vi "Send Message.vi"(0 "message queue in":T3, 1 "receiver port (0)":u16, 5 "message":T1, 9 "timeout (-1 ms)":i32=-1, 11 "error in":errorcluster) -> (4 "message queue out":T3, 10 "timed out?":bool, 15 "error out":errorcluster)   [LabVIEW 2015, in "Car Wash.lvlib" / "AMC.lvlib"]
doc: "Adds a message to:\n- the local queue passed in by reference if \"receiver host\" and \"receiver process\" are left undefined\n- another message queue on the local target if \"receiver host\" is undefined, but \"receiver process\" is specified\n- the message dispatch queue in another application instance if the receiver host and process are specified.\n\nIf \"receiver port\" is undefined, this VI will attempt to use the default UDP port.\n\nIf \"priority message\" is True, the message will be added to the front of the message queue.\n\nIf \"acknowledge message\" is True and the message is sent to another application instance, the receiver will send a reply message with the name format of \"AMC_Ack\" and a value of <name>. If \"message queue in\" is undefined, no acknowledge message will be sent."
uses:
  AMC.lvlib
  Message Queue.ctl
  Message.ctl
  Tools/Keyed Array/KeyedArray.ctl
  Send Message to Local Process.vi
  Send Message to Current Process.vi
  Read Local Dispatcher Port.vi
  FG Dispatcher Status.vi
  Get Local Name and IP.vi
  Globals.vi
  Tools/Keyed Array/Tools_KeyedArray.lvlib
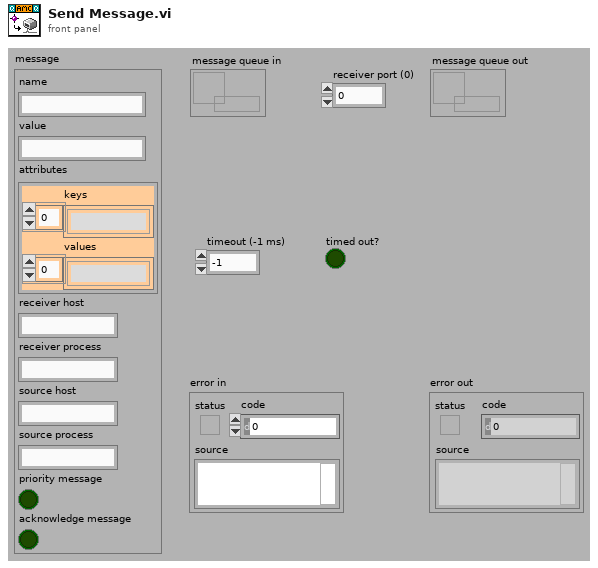
[diagram p1: front panel]
types:
  T1 = typedef "Car Wash.lvlib/AMC.lvlib/Message.ctl" = cluster{"name":string, "value":string, "attributes":T2, "receiver host":string, "receiver process":string, "source host":string, "source process":string, "priority message":bool, "acknowledge message":bool}
  T2 = typedef "Car Wash.lvlib/Tools_KeyedArray.lvlib/KeyedArray.ctl" = cluster{"keys":string[], "values":string[]}
  T3 = typedef "Car Wash.lvlib/AMC.lvlib/Message Queue.ctl" = refnum<queue>
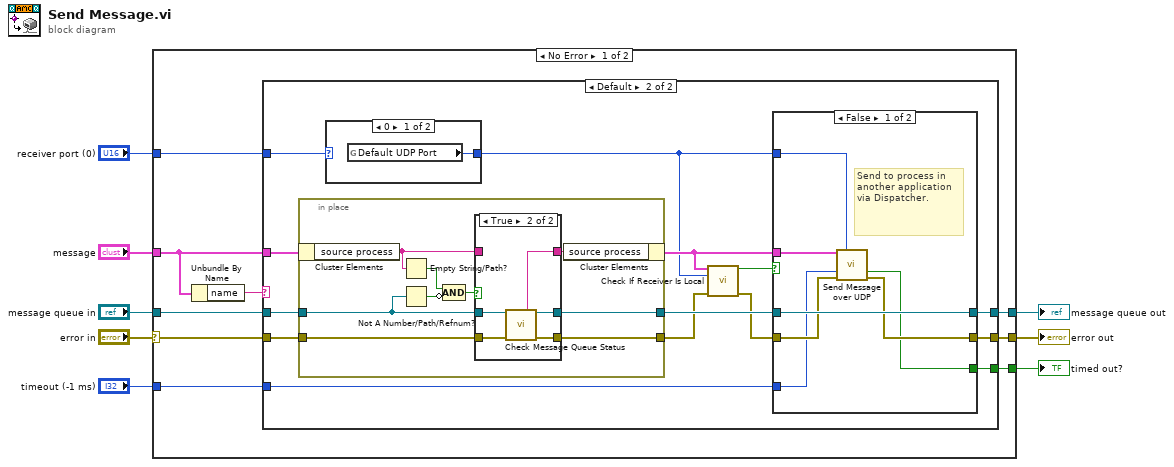
[diagram p0: block diagram]
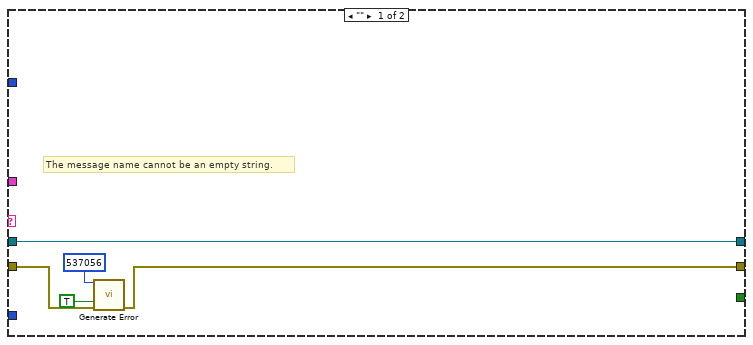
[diagram p2: hidden frame]
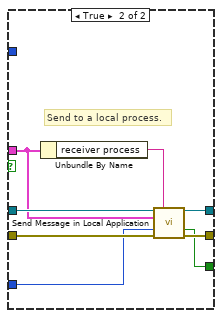
[diagram p5: hidden frame]
diagram:
  n1 = case shown="No Error" "error in" {
    selector: "error in" -> [w14 w71]
    tunnel: [w17 w71] -> w8
    tunnel: "message queue in" -> [w15 w72]
    tunnel: [w16 w72] -> w6
    tunnel: "message" -> [w10 _]
    tunnel: "timeout (-1 ms)" -> [w13 _]
    tunnel: [w12 _] -> w2
    tunnel: "receiver port (0)" -> [w11 _]
    frame No Error {
      n2 = Unbundle By Name(w10) -> ("name"=w9:string)
      n3 = case shown="Default" w9 {
        tunnel: [w19 w36] -> w17
        tunnel: [w22 w35] -> w16
        tunnel: w15 -> [w22 w34]
        tunnel: w14 -> [w20 w33]
        tunnel: w13 -> [_ w31]
        tunnel: [_ w30] -> w12
        tunnel: w11 -> [_ w25]
        tunnel: w10 -> [_ w23]
        frame "" {
          # "The message name cannot be an empty string."
          n4 = call "Generate Error.vi"("code"=537056, "status (F)"=TRUE, "error in"=w20) -> ("error out"=w19:errorcluster)  [unwired: 12 in]
        }
        frame Default {
          n5 = in-place {
            in-place-border: w34 -> [w42]
            in-place-border: w33 -> [w47]
            in-place-border: [w46] -> w32
            in-place-border: [w45] -> w26
            n6 = in-place-cluster #1(w23) -> ("source process"=w44:string)
            n7 = Empty String/Path?(string/path=w44) -> (empty?=w40:bool)
            n8 = Not A Number/Path/Refnum?(number/path/refnum=w42) -> (NaN/Path/Refnum?=w41:bool)
            n9 = Compound Arithmetic op=AND(w40, invert w41) -> (w39:bool)
            n10 = case shown="True" w39 {
              tunnel: w42 -> [w50 w55]
              tunnel: w47 -> [w49 w54]
              tunnel: [w50 w53] -> w46
              tunnel: [w49 w52] -> w45
              tunnel: [w48 w51] -> w43
              tunnel: w44 -> [w48 _]
              frame False {
              }
              frame True {
                n11 = call "Check Message Queue Status.vi"("message queue in"=w55, "error in"=w54) -> ("message queue name"=w51:string, "message queue out"=w53:T3, "error out"=w52:errorcluster)  [unwired: 9 in, 2 out]
              }
            }
            n12 = in-place-cluster #1("source process"=w43) -> (w28:T1)
          }
          n13 = case shown="0" w25 {
            selector: w25 -> [_ w38]
            tunnel: [w37 w38] -> w24
            frame 0 {
              n14 = global read "Globals.vi" "Default UDP Port"() -> (w37:u16)
            }
            frame Default {
            }
          }
          n15 = call "Check If Receiver Is Local.vi"("message"=w28, "UDP receiver port"=w24, "error in"=w26) -> ("local receiver?"=w29:bool, "error out"=w27:errorcluster)  [unwired: 11 in]
          n16 = case shown="False" w29 {
            tunnel: w27 -> [w60 w68]
            tunnel: [w61 w67] -> w36
            tunnel: w32 -> [w62 w70]
            tunnel: [w62 w69] -> w35
            tunnel: w28 -> [w56 w64]
            tunnel: w31 -> [w59 w66]
            tunnel: [w58 w65] -> w30
            tunnel: w24 -> [w57 _]
            frame False {
              # "Send to process in another application via Dispatcher."
              n17 = call "Send Message over UDP.vi"("message"=w56, "UDP receiver port"=w57, "timeout (25000 ms)"=w59, "error in"=w60) -> ("timed out?"=w58:bool, "error out"=w61:errorcluster)  [unwired: 9 in, 1 out]
            }
            frame True {
              # "Send to a local process."
              n18 = Unbundle By Name(w64) -> ("receiver process"=w63:string)
              n19 = call "Send Message in Local Application.vi"("message queue in"=w70, "receiver process (\"\" - local)"=w63, "message"=w64, "timeout (-1 ms)"=w66, "error in"=w68) -> ("message queue out"=w69:T3, "timed out?"=w65:bool, "error out"=w67:errorcluster)  [unwired: 8 in]
            }
          }
        }
      }
    }
    frame Error {
    }
  }
  "error out" <- w8
  "message queue out" <- w6
  "timed out?" <- w2
